vi "Cell tick.vi"(8 "error in (no error)":errorcluster, 11 "PlayerCell in":refnum<class "PlayerCell.lvclass">) -> (0 "error out":errorcluster, 3 "PlayerCell out":refnum<class "PlayerCell.lvclass">)   [LabVIEW 2019, in "PlayerCell.lvclass"]
uses:
  PlayerCell.lvclass
  Cell/Cell.lvclass
  Player/Player.lvclass
  Snake/Snake.lvclass
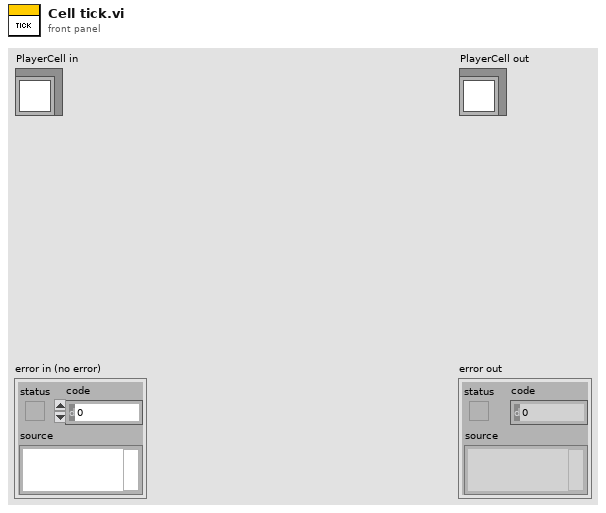
[diagram p1: front panel]
types:
  T1 = typedef "Direction STYP.ctl" = enum16{"Up", "Down", "Left", "Right"}
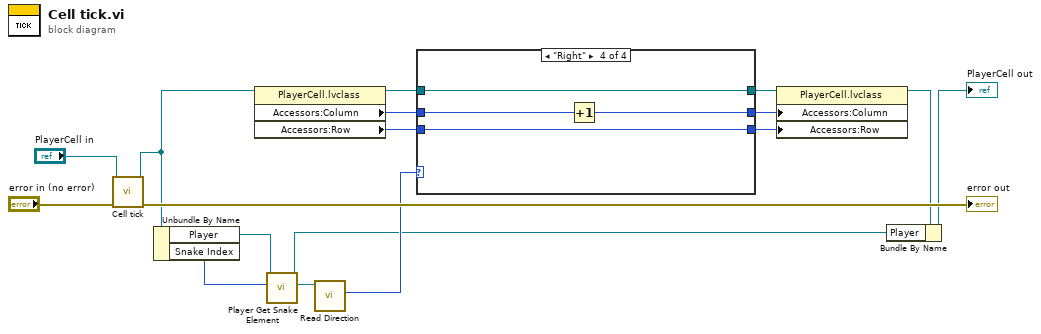
[diagram p0: block diagram]
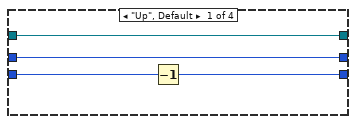
[diagram p2: hidden frame]
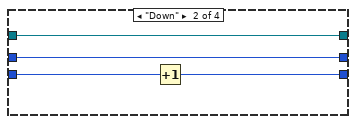
[diagram p3: hidden frame]
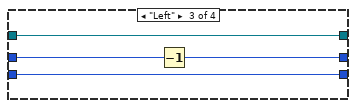
[diagram p4: hidden frame]
diagram:
  n1 = call-parent "Cell tick.vi"("error in (no error)"="error in (no error)", "Cell in"="PlayerCell in") -> ("error out"=→"error out":errorcluster, "Cell out"=w11:refnum<class "PlayerCell.lvclass">)  [unwired: 8 in]
  n2 = Unbundle By Name(w11) -> ("Player"=w14:refnum<class "Player.lvclass">, "Snake Index"=w13:i32)
  n3 = property class="PlayerCell.lvclass"(reference=w11) -> (reference out=w7:refnum<class "PlayerCell.lvclass">, "Accessors:Column"=w9:i32, "Accessors:Row"=w8:i32)  [unwired: 1 in, 1 out]
  n4 = call-dynamic "Player Get Snake Element.vi"("Index"=w13, "Player in"=w14) -> ("Snake"=w12:refnum<class "Snake.lvclass">, "Player out"=w1:refnum<class "Player.lvclass">)  [unwired: 7 in, 1 out]
  n5 = call-dynamic "Read Direction.vi"("Snake in"=w12) -> ("Direction"=w10:T1)  [unwired: 8 in, 2 out]
  n6 = case shown="\"Right\"" w10 {
    tunnel: w9 -> [w20 w24 w28 w32]
    tunnel: w8 -> [w19 w23 w27 w31]
    tunnel: w7 -> [w21 w25 w29 w33]
    tunnel: [w21 w25 w29 w33] -> w6
    tunnel: [w20 w24 w26 w30] -> w5
    tunnel: [w18 w22 w27 w31] -> w4
    frame "Up", Default {
      n7 = Decrement(x=w19) -> (x-1=w18:i32)
    }
    frame "Down" {
      n8 = Increment(x=w23) -> (x+1=w22:i32)
    }
    frame "Left" {
      n9 = Decrement(x=w28) -> (x-1=w26:i32)
    }
    frame "Right" {
      n10 = Increment(x=w32) -> (x+1=w30:i32)
    }
  }
  n11 = property class="PlayerCell.lvclass"(reference=w6, "Accessors:Column"=w5, "Accessors:Row"=w4) -> (reference out=w3:refnum<class "PlayerCell.lvclass">)  [unwired: 1 in, 1 out]
  n12 = Bundle By Name(cluster=w3, "Player"=w1) -> (→"PlayerCell out":refnum<class "PlayerCell.lvclass">)
